vi "Get Data.vi"(8 "error in (no error)":errorcluster, 11 "DataGrid.lvlib:Abstract EVENT.lvclass":refnum<class "Abstract EVENT.lvclass">) -> (0 "error out":errorcluster, 1 "column":i32, 2 "row":i32, 3 "cell value":string)   [LabVIEW 2013, in "DataGrid.lvlib" / "CellValueChanged.lvclass"]
doc: "Converts the class data for cellValue into individual components of the grid"
uses:
  CellValueChanged.lvclass
  Abstract EVENT/Abstract EVENT.lvclass
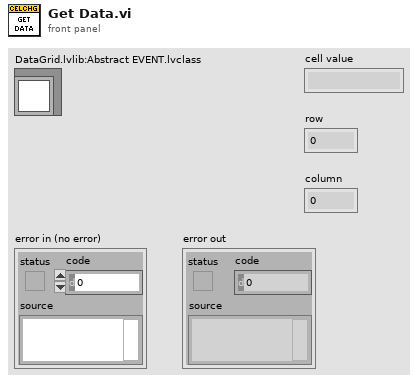
[diagram p1: front panel]
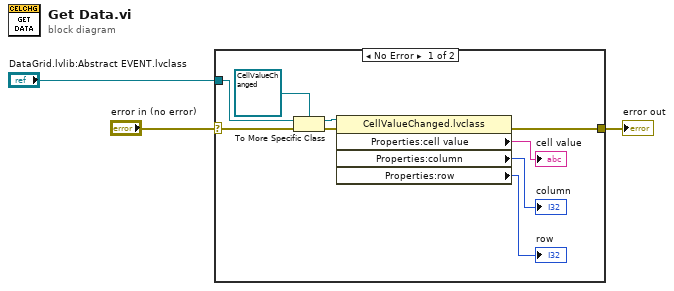
[diagram p0: block diagram]
diagram:
  n1 = case shown="No Error" "error in (no error)" {
    selector: "error in (no error)" -> [w5 w13]
    tunnel: [w12 w13] -> w2
    tunnel: "DataGrid.lvlib:Abstract EVENT.lvclass" -> [w7 _]
    frame No Error {
      n2 = To More Specific Class(target class=refnum<class "CellValueChanged.lvclass"> refnum ("DataGrid.lvlib:CellValueChanged.lvclass"), reference=w7, error in=w5) -> (specific class reference=w6:refnum<class "CellValueChanged.lvclass">, error out=w4:errorcluster)
      n3 = property class="CellValueChanged.lvclass"(reference=w6, error in=w4) -> (error out=w12:errorcluster, "Properties:cell value"=→"cell value":string, "Properties:column"=→"column":i32, "Properties:row"=→"row":i32)  [unwired: 1 out]
    }
    frame Error {
    }
  }
  "error out" <- w2
